vi "createSetForceFrame.vi"(0 "FAILC in":refnum<class "FAILC.lvclass">, 5 "WaitForTrigger":bool, 7 "TriggerIRQ":bool, 9 "SlewFlag":bool, 11 "error in (no error)":errorcluster) -> (4 "FAILC out":refnum<class "FAILC.lvclass">, 6 "Frame":T1 {"Data" format="%02x"}, 15 "error out":errorcluster)   [LabVIEW 2016, in "RTFAILC.lvlib" / "FAILC.lvclass"]
uses:
  FAILC.lvclass
  Common_RT_Modbus/DataTypes/Frame.ctl
  Common_RT_Modbus/RTModbus.lvlib
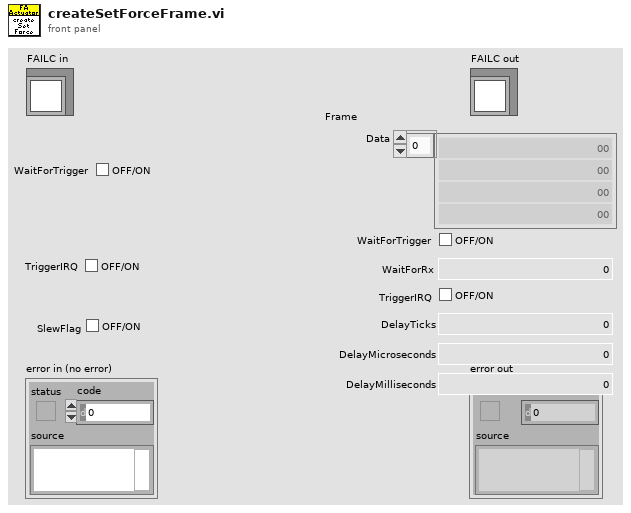
[diagram p1: front panel]
types:
  T1 = typedef "RTModbus.lvlib/Frame.ctl" = cluster{"Data":u8[], "WaitForTrigger":bool, "WaitForRx":u16, "TriggerIRQ":bool, "DelayTicks":u16, "DelayMicroseconds":u16, "DelayMilliseconds":u16}
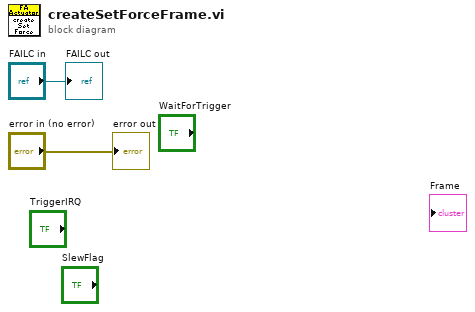
[diagram p0: block diagram]
diagram:
  "error out" <- "error in (no error)"
  "FAILC out" <- "FAILC in"
